vi "VI Tree1.vi"   [LabVIEW 2015, in "Agilent 3446X Series1.lvlib"]
doc: "This is the instrument driver for the Agilent 3446X Series. The VI Tree displays all the user-callable VIs of the instrument driver in an organized table."
uses:
  Agilent 3446X Series1.lvlib
  Data/Read (Single Point)1.vi
panel:
  # "(c) 2013 National Instruments.  ALL RIGHTS RESERVED."
  # "SEE DIAGRAM\nFOR VI TREE."
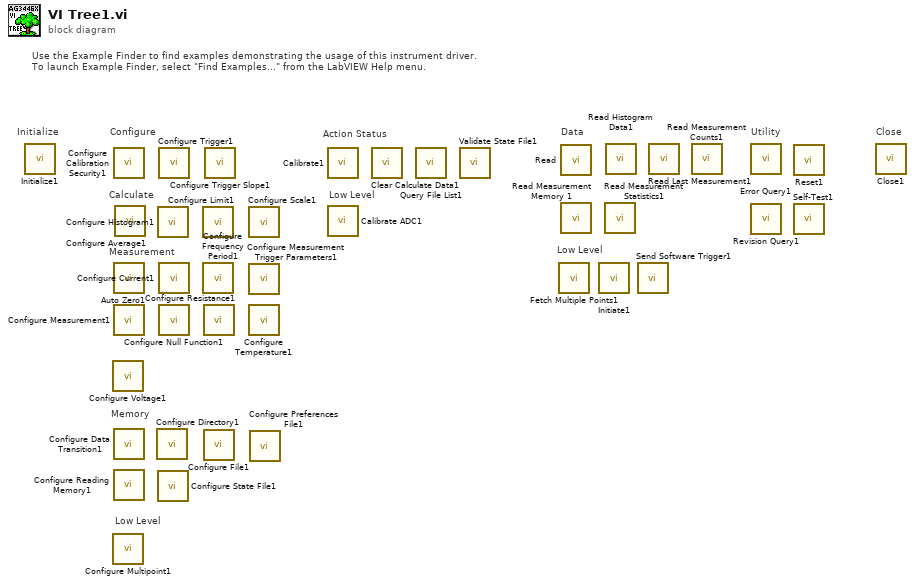
[diagram p0: block diagram]
diagram:
  # "Memory"
  # "Measurement"
  # "Calculate"
  # "Low Level"
  # "Action Status"
  # "Low Level"
  # "Low Level"
  # "Use the Example Finder to find examples demonstrating the usage of this instrument driver.\nTo launch Example Finder, select \"Find Examples...\" from the LabVIEW Help menu."
  # "Configure"
  # "Utility"
  # "Data"
  # "Close"
  # "Initialize"
  n1 = call "Initialize1.vi"() -> ()  [unwired: 9 in, 3 out]
  n2 = call "Configure Voltage1.vi"() -> ()  [unwired: 10 in, 2 out]
  n3 = call "Configure Multipoint1.vi"() -> ()  [unwired: 10 in, 2 out]
  n4 = call "Configure Calibration Security1.vi"() -> ()  [unwired: 10 in, 2 out]
  n5 = call "Auto Zero1.vi"() -> ()  [unwired: 10 in, 2 out]
  n6 = call "Configure Measurement1.vi"() -> ()  [unwired: 10 in, 2 out]
  n7 = call "Configure Data Transition1.vi"() -> ()  [unwired: 10 in, 2 out]
  n8 = call "Configure Reading Memory1.vi"() -> ()  [unwired: 10 in, 2 out]
  n9 = call "Configure Average1.vi"() -> ()  [unwired: 10 in, 2 out]
  n10 = call "Configure Directory1.vi"() -> ()  [unwired: 10 in, 2 out]
  n11 = call "Configure Histogram1.vi"() -> ()  [unwired: 10 in, 2 out]
  n12 = call "Configure State File1.vi"() -> ()  [unwired: 10 in, 2 out]
  n13 = call "Configure Trigger1.vi"() -> ()  [unwired: 10 in, 2 out]
  n14 = call "Configure Current1.vi"() -> ()  [unwired: 10 in, 2 out]
  n15 = call "Configure Null Function1.vi"() -> ()  [unwired: 10 in, 2 out]
  n16 = call "Configure Limit1.vi"() -> ()  [unwired: 10 in, 2 out]
  n17 = call "Configure Frequency Period1.vi"() -> ()  [unwired: 10 in, 2 out]
  n18 = call "Configure Resistance1.vi"() -> ()  [unwired: 10 in, 2 out]
  n19 = call "Configure File1.vi"() -> ()  [unwired: 10 in, 2 out]
  n20 = call "Configure Trigger Slope1.vi"() -> ()  [unwired: 10 in, 2 out]
  n21 = call "Configure Scale1.vi"() -> ()  [unwired: 10 in, 2 out]
  n22 = call "Configure Measurement Trigger Parameters1.vi"() -> ()  [unwired: 10 in, 2 out]
  n23 = call "Configure Temperature1.vi"() -> ()  [unwired: 10 in, 2 out]
  n24 = call "Configure Preferences File1.vi"() -> ()  [unwired: 10 in, 2 out]
  n25 = call "Calibrate1.vi"() -> ()  [unwired: 9 in, 3 out]
  n26 = call "Calibrate ADC1.vi"() -> ()  [unwired: 9 in, 3 out]
  n27 = call "Clear Calculate Data1.vi"() -> ()  [unwired: 10 in, 2 out]
  n28 = call "Query File List1.vi"() -> ()  [unwired: 7 in, 5 out]
  n29 = call "Validate State File1.vi"() -> ()  [unwired: 9 in, 3 out]
  n30 = call "Fetch Multiple Points1.vi"() -> ()  [unwired: 9 in, 3 out]
  n31 = call-poly "Read.vi"() -> ()  [unwired: 9 in, 3 out]
  n32 = call "Read Measurement Memory 1.vi"() -> ()  [unwired: 9 in, 3 out]
  n33 = call "Initiate1.vi"() -> ()  [unwired: 10 in, 2 out]
  n34 = call "Read Measurement Statistics1.vi"() -> ()  [unwired: 8 in, 8 out]
  n35 = call "Read Histogram Data1.vi"() -> ()  [unwired: 9 in, 3 out]
  n36 = call "Send Software Trigger1.vi"() -> ()  [unwired: 10 in, 2 out]
  n37 = call "Read Last Measurement1.vi"() -> ()  [unwired: 9 in, 3 out]
  n38 = call "Read Measurement Counts1.vi"() -> ()  [unwired: 9 in, 3 out]
  n39 = call "Error Query1.vi"() -> ()  [unwired: 8 in, 4 out]
  n40 = call "Revision Query1.vi"() -> ()  [unwired: 8 in, 4 out]
  n41 = call "Reset1.vi"() -> ()  [unwired: 10 in, 2 out]
  n42 = call "Self-Test1.vi"() -> ()  [unwired: 8 in, 4 out]
  n43 = call "Close1.vi"() -> ()  [unwired: 11 in, 1 out]
